vi "nano-positioner.vi"() -> ()   [LabVIEW 2014]
uses:
  <vilib>/Utility/inputDevices.llb/keyboardAcquire.vi
  <userlib>/Madlib/Madlib.dll
panel:
  in  "?":bool
  in  "Motion Multiplier":dbl(slide)=1.0 scale=1.0..100.0
  in  "Command rate":u16(ring)=10 items=["500 Hertz"=2, "100 Hertz"=10, "10 Hertz"=100, "1 Hertz"=1000]
  out "First Key":T1(ring)
  in  "Max Velocity":string(combo)="22"
  in  "Z Decreasing":string(combo)="21"
  in  "Z Increasing":string(combo)="24"
  in  "X Increasing":string(combo)="32"
  in  "X Decreasing":string(combo)="28"
  in  "Y Decreasing":string(combo)="10"
  in  "Y Increasing":string(combo)="13"
  out "Z (mM)":dbl format="%.3f"
  out "Y (mM)":dbl format="%.3g"
  out "X (mM)":dbl format="%.3f"
  out "Z Range (mM)":dbl
  out "Y Range (mM)":dbl
  out "X Range (mM)":dbl
  # "Command Rate"
  # "Key Configuration"
  # "Motion Multiplier"
  # "x1"
  # "x100"
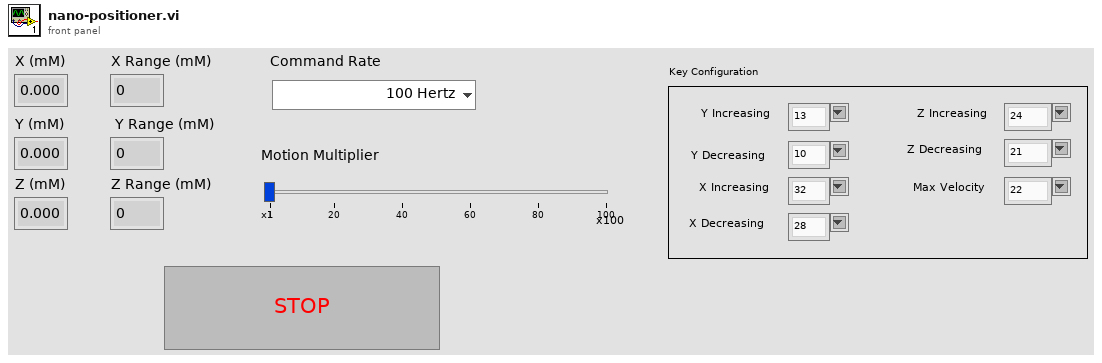
[diagram p1: front panel]
types:
  T1 = enum16{"0", "1", "2", "3", "4", "5", "6", "7", "8", "9", "A", "B", "C", "D", "E", "F", "G", "H", "I", "J", "K", "L", "M", "N", "O", "P", "Q", "R", "S", "T", "U", "V", "W", "X", "Y", "Z", "F1", "F2", "F3", "F4", "F5", "F6", "F7", "F8", "F9", "F10", "F11", "F12", "F13", "F14", "F15", "ADD", "BACK", "BACKSLASH", "CAPITAL", "COMMA", "DECIMAL", "DELETE", "DIVIDE", "DOWN", "END", "EQUALS", "ESCAPE", "GRAVE (`)", "HOME", "INSERT", "LBRACKET", "LCONTROL", "LEFT", "L ALT", "LSHIFT", "LWIN", "MINUS", "MULTIPLY", "NEXT", "NUMLOCK", "NUMPAD_0", "NUMPAD_1", "NUMPAD_2", "NUMPAD_3", "NUMPAD_4", "NUMPAD_5", "NUMPAD_6", "NUMPAD_7", "NUMPAD_8", "NUMPAD_9", "PAUSE", "PERIOD", "PRIOR (PG UP)", "RBRACKET", "RCONTROL", "RETURN", "RIGHT", "R ALT", "RSHIFT", "RWIN", "SCROLL", "SEMICOLON", "SLASH", "SPACE", "SUBTRACT", "TAB", "UP", "ENTER (num pad)", "' (quote)"}
  T2 = cluster{"X Command":dbl, "Y Command":dbl, "Z Command":dbl, "X Position":dbl, "Y Position":dbl, "Z Position":dbl, "X Calibration":dbl, "Y Calibration":dbl, "Z Calibration":dbl}
  T3 = cluster{"X Command":dbl, "Y Command":dbl, "Z Command":dbl, "X Position":dbl, "Y Position":dbl, "Z Position":dbl}
  T4 = enum16{"0", "1", "2", "3", "4", "5", "6", "7", "8", "9", "A", "B", "C", "D", "E", "F", "G", "H", "I", "J", "K", "L", "M", "N", "O", "P", "Q", "R", "S", "T", "U", "V", "W", "X", "Y", "Z", "F1", "F2", "F3", "F4", "F5", "F6", "F7", "F8", "F9", "F10", "F11", "F12", "F13", "F14", "F15", "ADD", "BACK", "BACKSLASH", "CAPITAL", "COMMA", "DECIMAL", "DELETE", "DIVIDE", "DOWN", "END", "EQUALS", "ESCAPE", "GRAVE (`)", "HOME", "INSERT", "LBRACKET", "LCONTROL", "LEFT", "L ALT", "LSHIFT", "LWIN", "MINUS", "MULTIPLY", "NEXT", "NUMLOCK", "NUMPAD_0", "NUMPAD_1", "NUMPAD_2", "NUMPAD_3", "NUMPAD_4", "NUMPAD_5", "NUMPAD_6", "NUMPAD_7", "NUMPAD_8", "NUMPAD_9", "PAUSE", "PERIOD", "PRIOR (PG UP)", "RBRACKET", "RCONTROL", "RETURN", "RIGHT", "R ALT", "RSHIFT", "RWIN", "SCROLL", "SEMICOLON", "SLASH", "SPACE", "SUBTRACT", "TAB", "UP", "ENTER (num pad)", "' (quote)"}[]
  T5 = cluster{"Y Increasing":string, "Y Decreasing":string, "X Increasing":string, "X Decreasing":string, "Z Increasing":string, "Z Decreasing":string, "Max Velocity":string}
  T6 = cluster{"X Command":dbl, "Y Command":dbl, "Z Command":dbl, "X Position":dbl, "Y Position":dbl, "position":dbl}
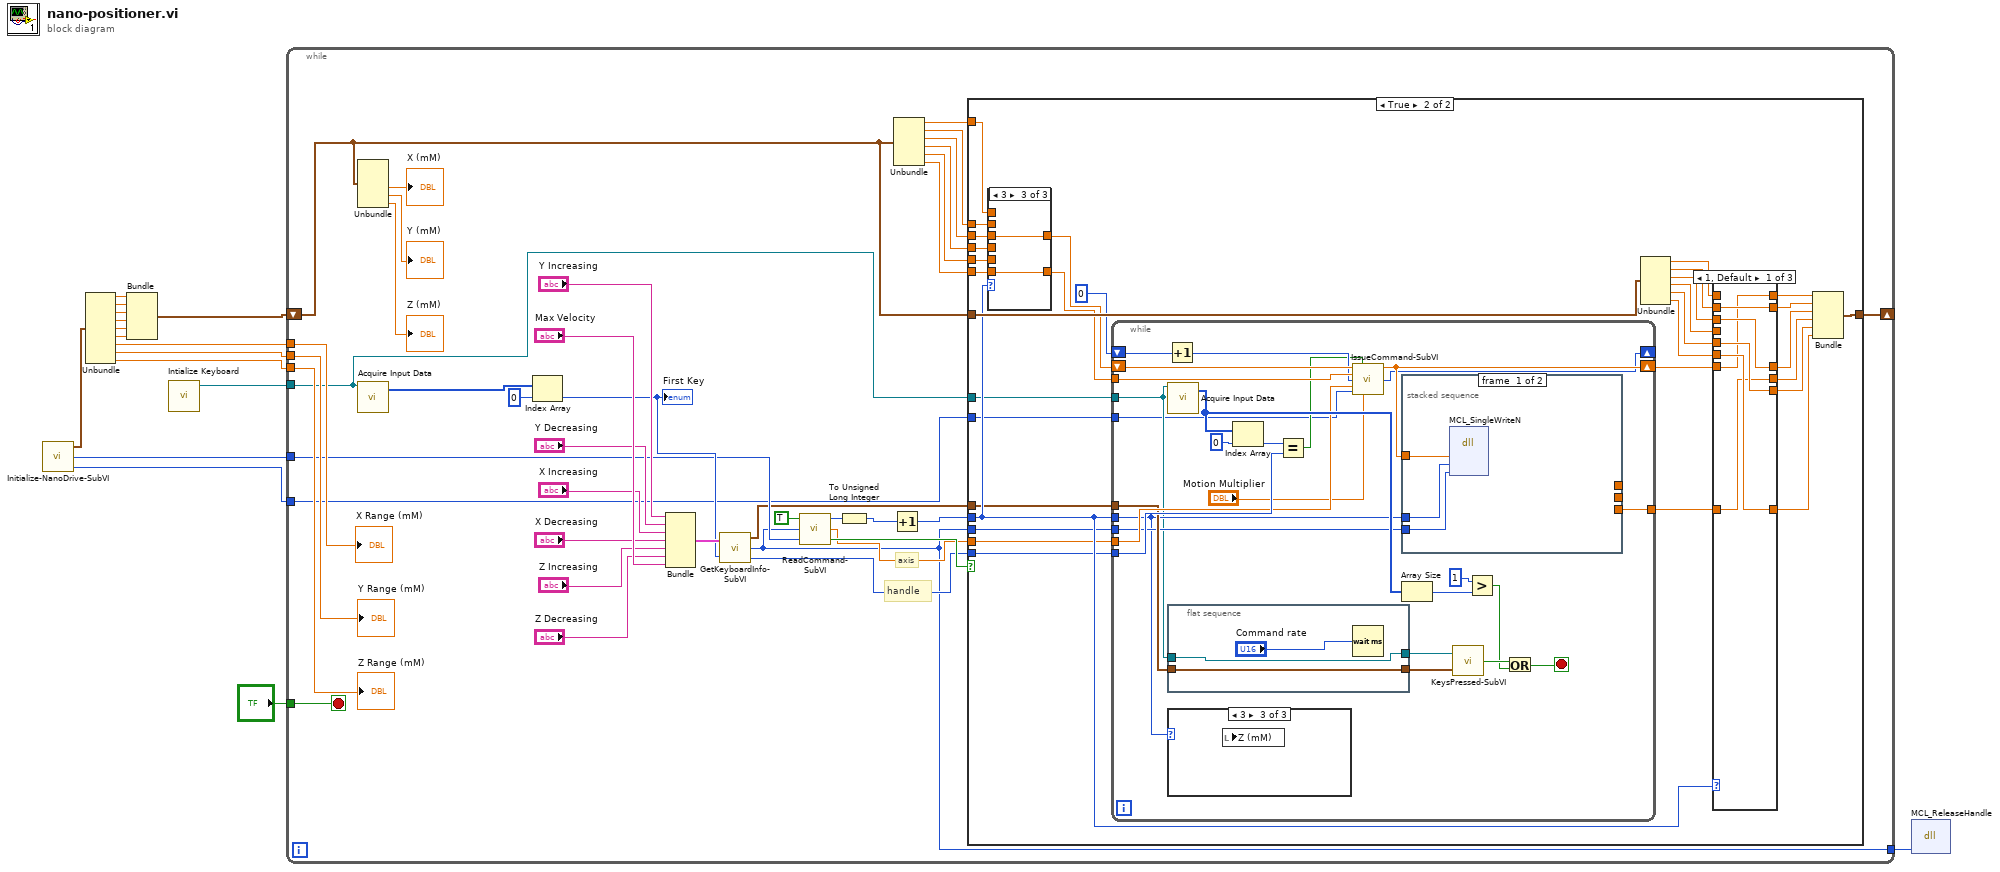
[diagram p0: block diagram]
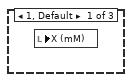
[diagram p5: hidden frame]
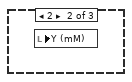
[diagram p6: hidden frame]
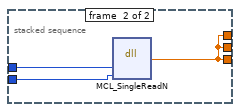
[diagram p7: hidden frame]
diagram:
  n1 = call "Initialize-NanoDrive-SubVI.vi"() -> ("Output Pos Info"=w16:T2, "Handle"=w4:i32, "ADC/DAC Resolution"=w3:u32)  [unwired: 1 in]
  n2 = Unbundle(w16) -> ("X Command"=w12:dbl, "Y Command"=w11:dbl, "Z Command"=w10:dbl, "X Position"=w9:dbl, "Y Position"=w8:dbl, "Z Position"=w7:dbl, "X Calibration"=w15:dbl, "Y Calibration"=w14:dbl, "Z Calibration"=w13:dbl)
  n3 = Bundle("X Command"=w12, "Y Command"=w11, "Z Command"=w10, "X Position"=w9, "Y Position"=w8, "Z Position"=w7) -> (w6:T3)  [unwired: 1 in]
  n4 = call <vilib>:"Intialize Keyboard.vi"() -> ("device ID"=w5:refnum<k1>)  [unwired: 1 in, 10 out]
  n5 = while {
    tunnel: w15 -> [w54]
    tunnel: w14 -> [w53]
    tunnel: w13 -> [w52]
    tunnel: w5 -> [w21]
    tunnel: w4 -> [w35]
    tunnel: w3 -> [w20]
    tunnel: "?" -> [w19]
    tunnel: [w18] -> w1
    shift-right: [w17] -> _
    shift-left: w6 -> [w48]
    stop <- w19 stop-if-true
    # "handle"
    # "axis"
    n6 = Unbundle(w48) -> ("X Position"=→"X (mM)":dbl, "Y Position"=→"Y (mM)":dbl, "Z Position"=→"Z (mM)":dbl)  [unwired: 3 out]
    n7 = call-poly <vilib>:"Acquire Input Data.vi"("device ID"=w21) -> ("keys pressed"=w39:T4)  [unwired: 1 in, 17 out]
    n8 = Index Array "Index Array"(array=w39, index=0) -> (element=w37:T1)
    "First Key" <- w37
    n9 = Bundle("Y Increasing"="Y Increasing", "Y Decreasing"="Y Decreasing", "X Increasing"="X Increasing", "X Decreasing"="X Decreasing", "Z Increasing"="Z Increasing", "Z Decreasing"="Z Decreasing", "Max Velocity"="Max Velocity") -> (w40:T5)  [unwired: 1 in]
    n10 = call "GetKeyboardInfo-SubVI.vi"("Key Selections"=w40, "Key\nValue"=w37) -> ("Key values"=w22:cluster{i32, i32, i32, i32, i32, i32, i32}, "number"=w18:u32, "Max Velocity Value"=w24:i32)
    n11 = call "ReadCommand-SubVI.vi"("handle"=w35, "Motion #"=w18, "Enable\n(True)"=TRUE) -> ("Enable Move\n(TRUE)"=w34:bool, "Direction"=w23:dbl, "Axis"=w33:enum16{"X", "Y", "Z"})
    n12 = To Unsigned Long Integer(number=w33) -> (unsigned 32bit integer=w32:u32)
    n13 = Increment(x=w32) -> (x+1=w31:u32)
    n14 = Unbundle(w48) -> ("X Command"=w29:dbl, "Y Command"=w28:dbl, "Z Command"=w26:dbl, "X Position"=w30:dbl, "Y Position"=w27:dbl, "Z Position"=w25:dbl)
    n15 = case shown="True" w34 {
      tunnel: w48 -> [w55 w87]
      tunnel: w31 -> [_ w65]
      tunnel: w30 -> [_ w86]
      tunnel: w29 -> [_ w85]
      tunnel: w28 -> [_ w82]
      tunnel: w27 -> [_ w81]
      tunnel: w26 -> [_ w80]
      tunnel: w25 -> [_ w79]
      tunnel: w24 -> [_ w64]
      tunnel: w23 -> [_ w63]
      tunnel: w22 -> [_ w62]
      tunnel: w21 -> [_ w61]
      tunnel: w18 -> [_ w60]
      tunnel: w20 -> [_ w58]
      tunnel: [w55 w56] -> w17
      frame False {
      }
      frame True {
        n16 = case shown="3" w65 {
          tunnel: [w89 w90 w92] -> w83
          tunnel: w86 -> [w89 _ _]
          tunnel: w85 -> [w88 _ _]
          tunnel: [w88 w91 w93] -> w84
          tunnel: w82 -> [_ w91 _]
          tunnel: w81 -> [_ w90 _]
          tunnel: w80 -> [_ _ w93]
          tunnel: w79 -> [_ _ w92]
          frame 1, Default {
          }
          frame 2 {
          }
          frame 3 {
          }
        }
        n17 = while {
          tunnel: w83 -> [w118]
          tunnel: w65 -> [w99]
          tunnel: w64 -> [w111]
          tunnel: w63 -> [w110]
          tunnel: w62 -> [w107]
          tunnel: w61 -> [w97]
          tunnel: w60 -> [w100]
          tunnel: [w98] -> w59
          tunnel: w58 -> [w96]
          shift-right: [w95] -> w57
          shift-left: w84 -> [w119]
          shift-right: [w94] -> _
          shift-left: 0 -> [w117]
          stop <- w101 stop-if-true
          n18 = Increment(x=w117) -> (x+1=w116:i32)
          n19 = call-poly <vilib>:"Acquire Input Data.vi"("device ID"=w97) -> ("keys pressed"=w114:T4)  [unwired: 1 in, 17 out]
          n20 = flat-sequence {
            tunnel: [w127] -> w109
            tunnel: w97 -> [w127]
            tunnel: [w126] -> w108
            tunnel: w107 -> [w126]
            frame #0 {
              n21 = Wait (ms)(milliseconds to wait="Command rate") -> ()  [unwired: 1 out]
            }
          }
          n22 = case shown="3" w99 {
            frame 1, Default {
              n23 = local read "X (mM)"() -> ()  [unwired: 1 in]
            }
            frame 2 {
              n24 = local read "Y (mM)"() -> ()  [unwired: 1 in]
            }
            frame 3 {
              n25 = local read "Z (mM)"() -> ()  [unwired: 1 in]
            }
          }
          n26 = Index Array(array=w114, index=0) -> (element=w113:T1)
          n27 = Equal?(x=w113, y=w111) -> (x = y?=w112:bool)
          n28 = call "IssueCommand-SubVI.vi"("Current Position"=w119, "Max Velocity?"=w112, "Calibration"=w118, "Loop Iteration"=w116, "Direction"=w110, "ADC/DAC Resolution"=w96, "Motion Multiplier"="Motion Multiplier") -> ("Pos. Command"=w95:dbl, "Loop Iteration Out"=w94:i32)  [unwired: 7 in]
          n29 = stacked-sequence {
            tunnel: w100 -> [w122 w124]
            tunnel: w99 -> [w121 w125]
            tunnel: [_ w123] -> _
            tunnel: w95 -> [w120 _]
            tunnel: [_ w123] -> _
            tunnel: [_ w123] -> w98
            frame #0 {
              n30 = dll-call lib="C:/Program Files (x86)/National Instruments/LabVIEW 2014/user.lib/Madlib/Madlib.dll" fn="MCL_SingleWriteN" label="Madlib.dll\nMCL_SingWriteN"("position"=w120, "axis"=w121, "handle"=w122) -> ()  [unwired: 6 in, 3 out]
            }
            frame #1 {
              n31 = dll-call lib="C:/Program Files (x86)/National Instruments/LabVIEW 2014/user.lib/Madlib/Madlib.dll" fn="MCL_SingleReadN" label="Madlib.dll:\nMCL_SingleReadN"("Axis"=w125, "Handle"=w124) -> ("position"=w123:dbl)  [unwired: 5 in, 2 out]
            }
          }
          n32 = Array Size(array=w114) -> (size(s)=w105:i32)
          n33 = call "KeysPressed-SubVI.vi"("Key values"=w108, "device ID"=w109) -> ("Stop = TRUE"=w103:bool)
          n34 = Greater?(x=1, y=w105) -> (0:w102:bool)
          n35 = Or(x=w103, y=w102) -> (x .or. y?=w101:bool)
        }
        n36 = Unbundle(w87) -> ("X Command"=w78:dbl, "Y Command"=w77:dbl, "Z Command"=w76:dbl, "X Position"=w75:dbl, "Y Position"=w74:dbl, "Z Position"=w73:dbl)
        n37 = case shown="1, Default" w65 {
          tunnel: w78 -> [_ w140 w146]
          tunnel: w77 -> [w134 _ w145]
          tunnel: w76 -> [w133 w138 _]
          tunnel: w75 -> [_ w139 w144]
          tunnel: w74 -> [w132 _ w143]
          tunnel: w73 -> [w131 w137 _]
          tunnel: [w134 w135 w145] -> w72
          tunnel: [w133 w138 w141] -> w71
          tunnel: [w132 w136 w143] -> w69
          tunnel: [w131 w137 w142] -> w70
          tunnel: [w129 w140 w146] -> w68
          tunnel: [w130 w139 w144] -> w67
          tunnel: w59 -> [w130 w136 w142]
          tunnel: w57 -> [w129 w135 w141]
          frame 1, Default {
          }
          frame 2 {
          }
          frame 3 {
          }
        }
        n38 = Bundle("X Command"=w68, "Y Command"=w72, "Z Command"=w71, "X Position"=w67, "Y Position"=w69, "position"=w70) -> (w56:T6)  [unwired: 1 in]
      }
    }
    "X Range (mM)" <- w54
    "Y Range (mM)" <- w53
    "Z Range (mM)" <- w52
  }
  n39 = dll-call lib="C:/Program Files (x86)/National Instruments/LabVIEW 2014/user.lib/Madlib/Madlib.dll" fn="MCL_ReleaseHandle" label="Madlib.dll:\nMCL_ReleaseHandle"("handle"=w1) -> ()  [unwired: 4 in, 3 out]
